vi "Run Pure Pursuit.vi"(6 "Synchronication":enum16{"Start", "Wait"}(ring)=enum."Wait", 7 "Description":string, 8 "Command Info In":T1, 10 "Reverse? (F)":bool, 11 "Path":cluster{dbl, "interpolation value":dbl}[](array[cluster])) -> (0 "Command Info Out":T1)   [LabVIEW 2017]
doc: "This VI notifies the subsystem to perform this command for the given duration, then go back to the default state. Synchronization determines whether this VI Starts the operation and returns immediately, or waits for the operation to complete. The first option is commonly used for TeleOp, and the second for Autonomous sequencing."
uses:
  <vilib>/Rock Robotics/WPI/Framework/Command Status Info.ctl
  <vilib>/Rock Robotics/WPI/Framework/Completion Status.ctl
  <vilib>/Rock Robotics/WPI/Framework/Completion Notifier.ctl
  Implementation/Drive Setpoints.ctl
  Implementation/Drive Operations.ctl
  Auton/Auton Kill Switch.vi
  Pure Pursuit/Pure Pursuit.lvlib
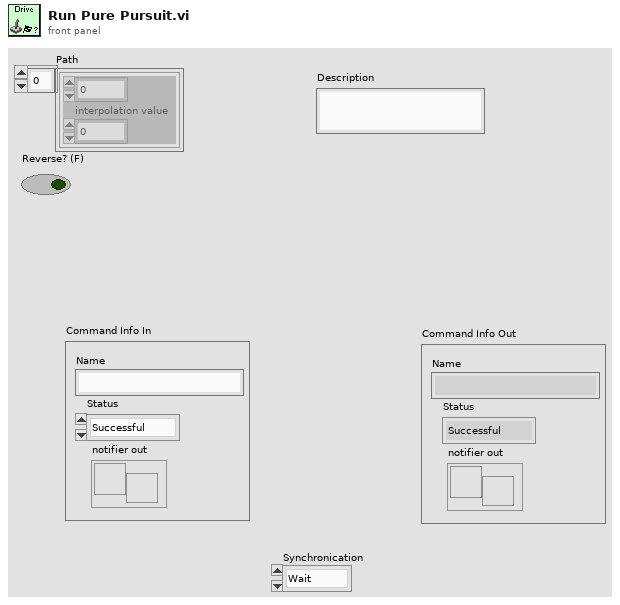
[diagram p1: front panel]
types:
  T1 = typedef "Command Status Info.ctl" = cluster{"Name":string, "Status":T2, "notifier out":T3}
  T2 = typedef "Completion Status.ctl" = enum16{"Successful", "Aborted", "Incomplete"}
  T3 = typedef "Completion Notifier.ctl" = refnum<notifier>
  T4 = typedef "Drive Setpoints.ctl" = cluster{"Operation":T5, "Left Setpoint":dbl, "Right Setpoint":dbl, "Duration":dbl, "Data":variant}
  T5 = typedef "Drive Operations.ctl" = enum16{"Reserve", "Read Current", "Immediate", "Drive for Time", "Drive for Distance", "Turn to Angle", "Drivetrain Char", "Pure Pursuit"}
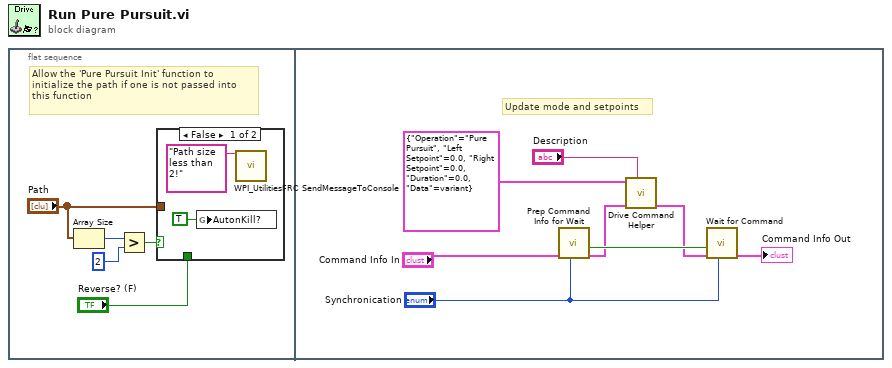
[diagram p0: block diagram]
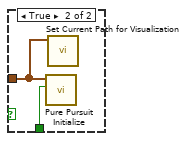
[diagram p2: hidden frame]
diagram:
  n1 = flat-sequence {
    frame #0 {
      # "Allow the 'Pure Pursuit Init' function to initialize the path if one is not passed into this function"
      n2 = Array Size(array="Path") -> (size(s)=w4:i32)
      n3 = Greater?(x=w4, y=2) -> (0:w3:bool)
      n4 = case shown="False" w3 {
        tunnel: "Path" -> [_ w9]
        tunnel: "Reverse? (F)" -> [_ w8]
        frame False {
          n5 = global write "Auton Kill Switch.vi" "AutonKill?"(TRUE ("AutonKill?")) -> ()
          n6 = call <vilib>:"WPI_UtilitiesFRC SendMessageToConsole.vi"("Message"="Path size less than 2!") -> ()  [unwired: 14 in, 1 out]
        }
        frame True {
          n7 = call "Pure Pursuit Initialize.vi"("Reverse? (F)"=w8, "Path"=w9) -> ()  [unwired: 9 in, 1 out]
          n8 = call "Set Current Path for Visualization.vi"("Path"=w9) -> ()  [unwired: 11 in]
        }
      }
    }
    frame #1 {
      # "Update mode and setpoints"
      n9 = call <vilib>:"Prep Command Info for Wait.vi"("Synchronication"="Synchronication", "Command Info"="Command Info In") -> ("Command Info"=w15:T1, "Allocated"=w16:bool)  [unwired: 8 in]
      n10 = call "Drive Command Helper.vi"("Description"="Description", "Command Info In"=w15, "SubSystem Data"=T4 {"Operation"=enum."Pure Pursuit", "Left Setpoint"=0.0, "Right Setpoint"=0.0, "Duration"=0.0, "Data"=variant}) -> ("Command Info Out"=w12:T1)  [unwired: 6 in, 2 out]
      n11 = call <vilib>:"Wait for Command.vi"("Synchronication"="Synchronication", "Command Info in"=w12, "Allocated"=w16) -> ("Command Info out"=→"Command Info Out":T1)  [unwired: 8 in]
    }
  }
